vi "06-RandomNumbers3.vi"() -> ()   [LabVIEW 2019]
panel:
  out "Less than 5":bool
  out "Greather than or equal to 5":bool
  out "Loop Count":dbl
  out "Random Number":dbl
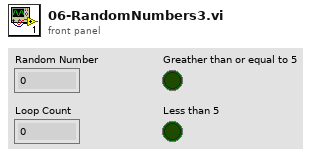
[diagram p1: front panel]
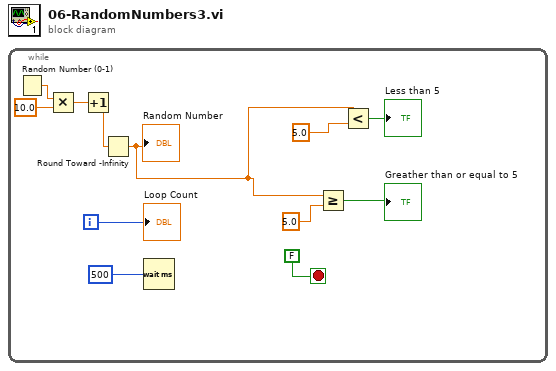
[diagram p0: block diagram]
diagram:
  n1 = while {
    i -> [w12]
    stop <- FALSE stop-if-true
    n2 = Random Number (0-1)() -> (number: 0 to 1=w9:dbl)
    n3 = Multiply(x=w9, y=10.0) -> (x*y=w7:dbl)
    n4 = Increment(x=w7) -> (x+1=w6:dbl)
    n5 = Round Toward -Infinity(1:w6) -> (0:w2:dbl)
    "Random Number" <- w2
    n6 = Wait (ms)(milliseconds to wait=u32 500) -> ()  [unwired: 1 out]
    n7 = Greater Or Equal?(x=w2, y=5.0) -> (x >= y?=→"Greather than or equal to 5":bool)
    n8 = Less?(x=w2, y=5.0) -> (x < y?=→"Less than 5":bool)
    "Loop Count" <- w12
  }
